vi "test Loopback MC with Start Stop and Status.vi"(8 "error in":errorcluster, 11 "TestCase in":refnum<class "Loopback.lvclass">) -> (0 "error out":errorcluster, 3 "TestCase out":refnum<class "Loopback.lvclass">)   [LabVIEW 2020, in "Loopback.lvclass"]
uses:
  Loopback.lvclass
  C:/dev/niveristand-custom-device-testing-tools/VeriStandTestCase/VeriStandTestCase.lvclass
  <vilib>/numeric/Random Number (Range) U64.vi
  485b7c2b-8320-4722-9ec7-d01f27c65546.vi
  cbc5c385-99ae-4ee9-9433-d6a44dd842bc.vi
  412f3c08-5d5c-44d4-ba0c-e78ba60fad11.vi
  849d8f76-503e-4f73-a17f-6140b744aaa7.vi
  0f9dda61-2c21-4955-8588-a8fc95227647.vi
  c1072d6c-53a2-4b9a-88af-ad4a91435edd.vi
  d6433e8a-b9d0-4f33-89c0-bfe3ca19b651.vi
  62366d90-b7ce-4d5b-90d7-fbdeef7ff138.vi
  <vilib>/numeric/sub_Random U32.vi
  <vilib>/NI VeriStand/Execution/Workspace/NI VeriStand - Set Single Channel Value.vi
  <vilib>/NI VeriStand/Execution/Workspace/NI VeriStand - Get Single Channel Value.vi
  <vilib>/NI VeriStand/Execution/Workspace/NI VeriStand - Get Multiple Channel Values.vi
  <vilib>/addons/_JKI Toolkits/VI Tester/TestCase.llb/TestCase.lvclass
  <vilib>/NI VeriStand/Execution/Workspace/NI_VS Workspace ExecutionAPI.lvlib
  C:/Program Files (x86)/National Instruments/LabVIEW 2020/vi.lib/addons/_JKI Toolkits/VI Tester/TestCase.llb/TestCase.lvclass
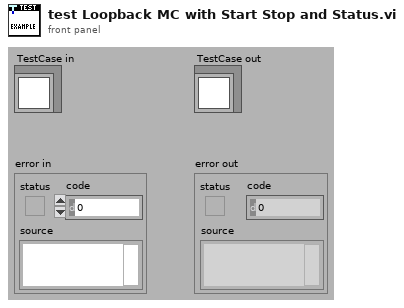
[diagram p1: front panel]
types:
  T1 = typedef "NI_VS Workspace ExecutionAPI.lvlib/WorkspaceAPI.ctl" = refnum<k24>
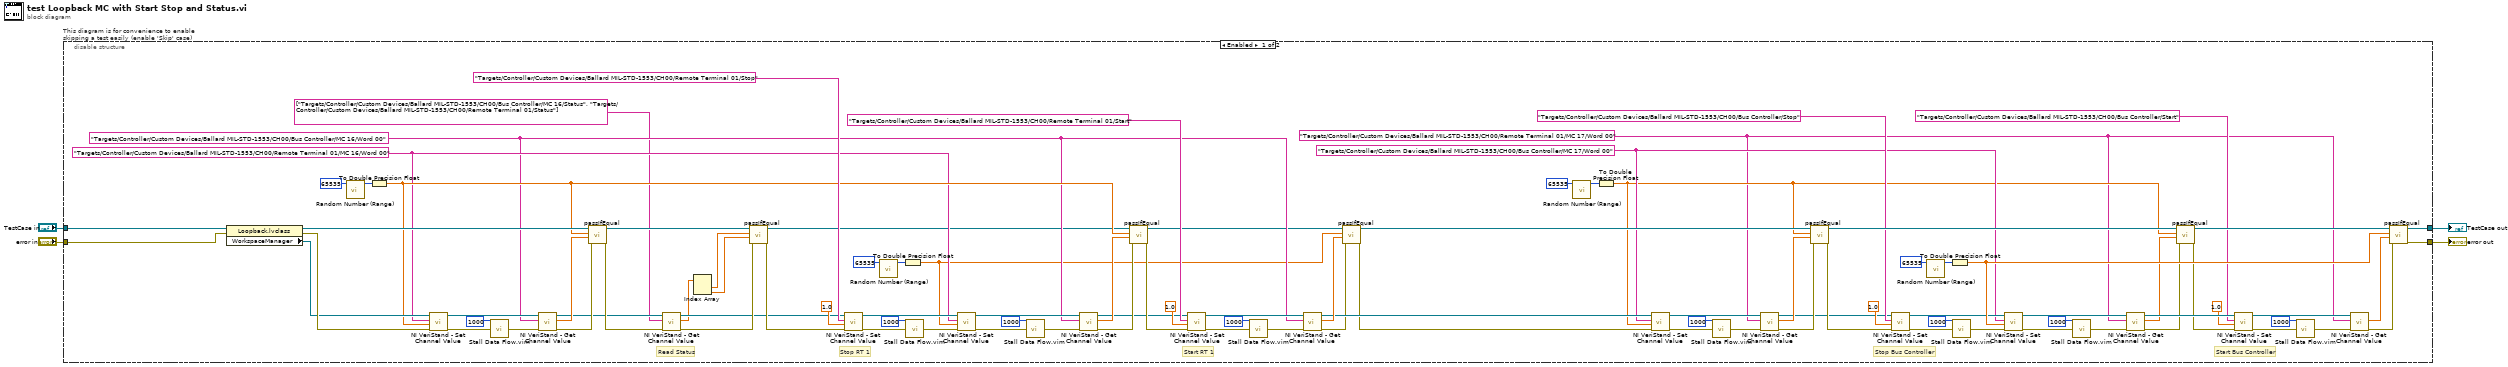
[diagram p0: block diagram]
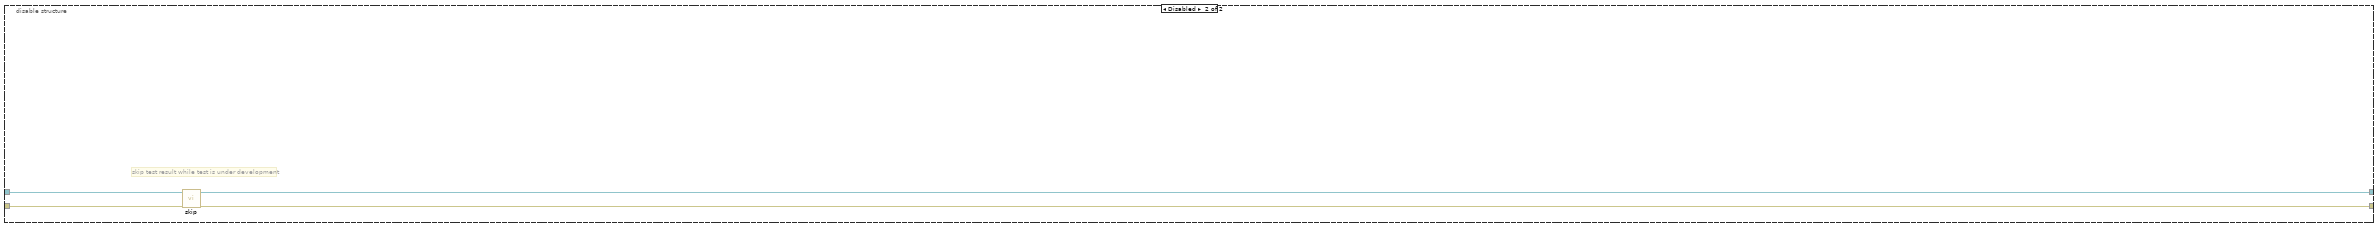
[diagram p2: hidden frame]
diagram:
  n1 = disable-structure "This diagram is for convenience to enable skipping a test easily (enable 'Skip' case)" shown="Enabled" {
    disable-tunnel: "TestCase in" -> [w93 w106]
    disable-tunnel: [w18 w104] -> w1
    disable-tunnel: [w17 w105] -> w3
    disable-tunnel: "error in" -> [w92 w103]
    frame Enabled {
      w19 = "Targets/Controller/Custom Devices/Ballard MIL-STD-1553/CH00/Remote Terminal 01/MC 17/Word 00" ("Channel")
      w22 = "Targets/Controller/Custom Devices/Ballard MIL-STD-1553/CH00/Bus Controller/MC 17/Word 00" ("Channel")
      w57 = "Targets/Controller/Custom Devices/Ballard MIL-STD-1553/CH00/Bus Controller/MC 16/Word 00" ("Channel")
      w71 = "Targets/Controller/Custom Devices/Ballard MIL-STD-1553/CH00/Remote Terminal 01/MC 16/Word 00" ("Channel")
      # "Read Status"
      # "Start Bus Controller"
      # "Stop Bus Controller"
      # "Start RT 1"
      # "Stop RT 1"
      n2 = property class="Loopback.lvclass"(reference=w93, error in=w92) -> (reference out=w102:refnum<class "Loopback.lvclass">, error out=w97:errorcluster, "WorkspaceManager"=w95:T1)
      n3 = call-poly <vilib>:"Random Number (Range).vi"("upper bound (100)"=u64 65535) -> ("number"=w85:u64)  [unwired: 10 in]
      n4 = To Double Precision Float(number=w85) -> (double precision float=w75:dbl)
      n5 = call-poly <vilib>:"NI VeriStand - Set Channel Value.vi"("error in (no error)"=w97, "Value"=w75, "Channel"=w71, "WorkspaceManager in"=w95) -> ("error out"=w99:errorcluster, "WorkspaceManager out"=w101:T1)  [unwired: 6 in]
      n6 = call "Stall Data Flow.vim"("value in"=w99, "milliseconds to wait"=u32 1000) -> ("value out"=w100:errorcluster)  [unwired: 1 out]
      n7 = call-poly <vilib>:"NI VeriStand - Get Channel Value.vi"("error in (no error)"=w100, "Channel"=w57, "WorkspaceManager in"=w101) -> ("error out"=w96:errorcluster, "Value"=w94:dbl, "WorkspaceManager out"=w12:T1)  [unwired: 6 in]
      n8 = call-dynamic "passIfEqual.vi"("error in (no error)"=w96, "y"=w94, "x"=w75, "TestCase in"=w102) -> ("error out"=w14:errorcluster, "TestCase out"=w13:refnum<class "Loopback.lvclass">)  [unwired: 6 in]
      n9 = call-poly <vilib>:"NI VeriStand - Get Channel Value.vi"("error in (no error)"=w14, "Channels"=string[] ["Targets/Controller/Custom Devices/Ballard MIL-STD-1553/CH00/Bus Controller/MC 16/Status", "Targets/Controller/Custom Devices/Ballard MIL-STD-1553/CH00/Remote Terminal 01/Status"], "WorkspaceManager in"=w12) -> ("error out"=w15:errorcluster, "Values"=w8:dbl[], "WorkspaceManager out"=w9:T1)  [unwired: 6 in]
      n10 = Index Array(array=w8) -> (element #1=w7:dbl, element #2=w6:dbl)  [unwired: 2 in]
      n11 = call-dynamic "passIfEqual.vi"("error in (no error)"=w15, "y"=w6, "x"=w7, "TestCase in"=w13) -> ("error out"=w10:errorcluster, "TestCase out"=w11:refnum<class "Loopback.lvclass">)  [unwired: 6 in]
      n12 = call-poly <vilib>:"NI VeriStand - Set Channel Value.vi"("error in (no error)"=w10, "Value"=1.0, "Channel"="Targets/Controller/Custom Devices/Ballard MIL-STD-1553/CH00/Remote Terminal 01/Stop", "WorkspaceManager in"=w9) -> ("error out"=w78:errorcluster, "WorkspaceManager out"=w73:T1)  [unwired: 6 in]
      n13 = call-poly <vilib>:"Random Number (Range).vi"("upper bound (100)"=u64 65535) -> ("number"=w66:u64)  [unwired: 10 in]
      n14 = To Double Precision Float(number=w66) -> (double precision float=w54:dbl)
      n15 = call "Stall Data Flow.vim"("value in"=w78, "milliseconds to wait"=u32 1000) -> ("value out"=w74:errorcluster)  [unwired: 1 out]
      n16 = call-poly <vilib>:"NI VeriStand - Set Channel Value.vi"("error in (no error)"=w74, "Value"=w54, "Channel"=w71, "WorkspaceManager in"=w73) -> ("error out"=w69:errorcluster, "WorkspaceManager out"=w72:T1)  [unwired: 6 in]
      n17 = call "Stall Data Flow.vim"("value in"=w69, "milliseconds to wait"=u32 1000) -> ("value out"=w68:errorcluster)  [unwired: 1 out]
      n18 = call-poly <vilib>:"NI VeriStand - Get Channel Value.vi"("error in (no error)"=w68, "Channel"=w57, "WorkspaceManager in"=w72) -> ("error out"=w80:errorcluster, "Value"=w81:dbl, "WorkspaceManager out"=w60:T1)  [unwired: 6 in]
      n19 = call-dynamic "passIfEqual.vi"("error in (no error)"=w80, "y"=w81, "x"=w75, "TestCase in"=w11) -> ("error out"=w62:errorcluster, "TestCase out"=w56:refnum<class "Loopback.lvclass">)  [unwired: 6 in]
      n20 = call-poly <vilib>:"NI VeriStand - Set Channel Value.vi"("error in (no error)"=w62, "Value"=1.0, "Channel"="Targets/Controller/Custom Devices/Ballard MIL-STD-1553/CH00/Remote Terminal 01/Start", "WorkspaceManager in"=w60) -> ("error out"=w64:errorcluster, "WorkspaceManager out"=w59:T1)  [unwired: 6 in]
      n21 = call "Stall Data Flow.vim"("value in"=w64, "milliseconds to wait"=u32 1000) -> ("value out"=w58:errorcluster)  [unwired: 1 out]
      n22 = call-poly <vilib>:"NI VeriStand - Get Channel Value.vi"("error in (no error)"=w58, "Channel"=w57, "WorkspaceManager in"=w59) -> ("error out"=w52:errorcluster, "Value"=w55:dbl, "WorkspaceManager out"=w53:T1)  [unwired: 6 in]
      n23 = call-dynamic "passIfEqual.vi"("error in (no error)"=w52, "y"=w55, "x"=w54, "TestCase in"=w56) -> ("error out"=w51:errorcluster, "TestCase out"=w50:refnum<class "Loopback.lvclass">)  [unwired: 6 in]
      n24 = call-poly <vilib>:"Random Number (Range).vi"("upper bound (100)"=u64 65535) -> ("number"=w83:u64)  [unwired: 10 in]
      n25 = To Double Precision Float(number=w83) -> (double precision float=w21:dbl)
      n26 = call-poly <vilib>:"NI VeriStand - Set Channel Value.vi"("error in (no error)"=w51, "Value"=w21, "Channel"=w22, "WorkspaceManager in"=w53) -> ("error out"=w88:errorcluster, "WorkspaceManager out"=w86:T1)  [unwired: 6 in]
      n27 = call "Stall Data Flow.vim"("value in"=w88, "milliseconds to wait"=u32 1000) -> ("value out"=w87:errorcluster)  [unwired: 1 out]
      n28 = call-poly <vilib>:"NI VeriStand - Get Channel Value.vi"("error in (no error)"=w87, "Channel"=w19, "WorkspaceManager in"=w86) -> ("error out"=w90:errorcluster, "Value"=w91:dbl, "WorkspaceManager out"=w16:T1)  [unwired: 6 in]
      n29 = call-dynamic "passIfEqual.vi"("error in (no error)"=w90, "y"=w91, "x"=w21, "TestCase in"=w50) -> ("error out"=w25:errorcluster, "TestCase out"=w24:refnum<class "Loopback.lvclass">)  [unwired: 6 in]
      n30 = call-poly <vilib>:"NI VeriStand - Set Channel Value.vi"("error in (no error)"=w25, "Value"=1.0, "Channel"="Targets/Controller/Custom Devices/Ballard MIL-STD-1553/CH00/Bus Controller/Stop", "WorkspaceManager in"=w16) -> ("error out"=w29:errorcluster, "WorkspaceManager out"=w32:T1)  [unwired: 6 in]
      n31 = call-poly <vilib>:"Random Number (Range).vi"("upper bound (100)"=u64 65535) -> ("number"=w38:u64)  [unwired: 10 in]
      n32 = To Double Precision Float(number=w38) -> (double precision float=w48:dbl)
      n33 = call "Stall Data Flow.vim"("value in"=w29, "milliseconds to wait"=u32 1000) -> ("value out"=w31:errorcluster)  [unwired: 1 out]
      n34 = call-poly <vilib>:"NI VeriStand - Set Channel Value.vi"("error in (no error)"=w31, "Value"=w48, "Channel"=w22, "WorkspaceManager in"=w32) -> ("error out"=w35:errorcluster, "WorkspaceManager out"=w33:T1)  [unwired: 6 in]
      n35 = call "Stall Data Flow.vim"("value in"=w35, "milliseconds to wait"=u32 1000) -> ("value out"=w36:errorcluster)  [unwired: 1 out]
      n36 = call-poly <vilib>:"NI VeriStand - Get Channel Value.vi"("error in (no error)"=w36, "Channel"=w19, "WorkspaceManager in"=w33) -> ("error out"=w27:errorcluster, "Value"=w26:dbl, "WorkspaceManager out"=w43:T1)  [unwired: 6 in]
      n37 = call-dynamic "passIfEqual.vi"("error in (no error)"=w27, "y"=w26, "x"=w21, "TestCase in"=w24) -> ("error out"=w42:errorcluster, "TestCase out"=w46:refnum<class "Loopback.lvclass">)  [unwired: 6 in]
      n38 = call-poly <vilib>:"NI VeriStand - Set Channel Value.vi"("error in (no error)"=w42, "Value"=1.0, "Channel"="Targets/Controller/Custom Devices/Ballard MIL-STD-1553/CH00/Bus Controller/Start", "WorkspaceManager in"=w43) -> ("error out"=w40:errorcluster, "WorkspaceManager out"=w44:T1)  [unwired: 6 in]
      n39 = call "Stall Data Flow.vim"("value in"=w40, "milliseconds to wait"=u32 1000) -> ("value out"=w45:errorcluster)  [unwired: 1 out]
      n40 = call-poly <vilib>:"NI VeriStand - Get Channel Value.vi"("error in (no error)"=w45, "Channel"=w19, "WorkspaceManager in"=w44) -> ("error out"=w49:errorcluster, "Value"=w47:dbl)  [unwired: 6 in, 1 out]
      n41 = call-dynamic "passIfEqual.vi"("error in (no error)"=w49, "y"=w47, "x"=w48, "TestCase in"=w46) -> ("error out"=w17:errorcluster, "TestCase out"=w18:refnum<class "Loopback.lvclass">)  [unwired: 6 in]
    }
    frame Disabled {
      # "skip test result while test is under development"
      n42 = call <vilib>:"skip.vi"("error in (no error)"=w103, "TestCase in"=w106) -> ("error out"=w105:errorcluster, "TestCase out"=w104:refnum<class "Loopback.lvclass">)  [unwired: 8 in]
    }
  }
  "error out" <- w3
  "TestCase out" <- w1
